vi "intersect circle.vi"(1 "max dist":dbl=40.0, 2 "R":dbl[](array[numeric]), 3 "Look":dbl(slide) scale=3.2..-3.2, 4 "R pos":dbl[](array[numeric]), 5 "py":dbl[](array[numeric]), 6 "px":dbl[](array[numeric])) -> (0 "Dist":dbl)   [LabVIEW 2009]
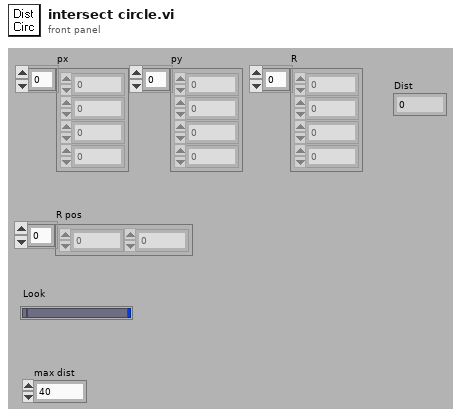
[diagram p1: front panel]
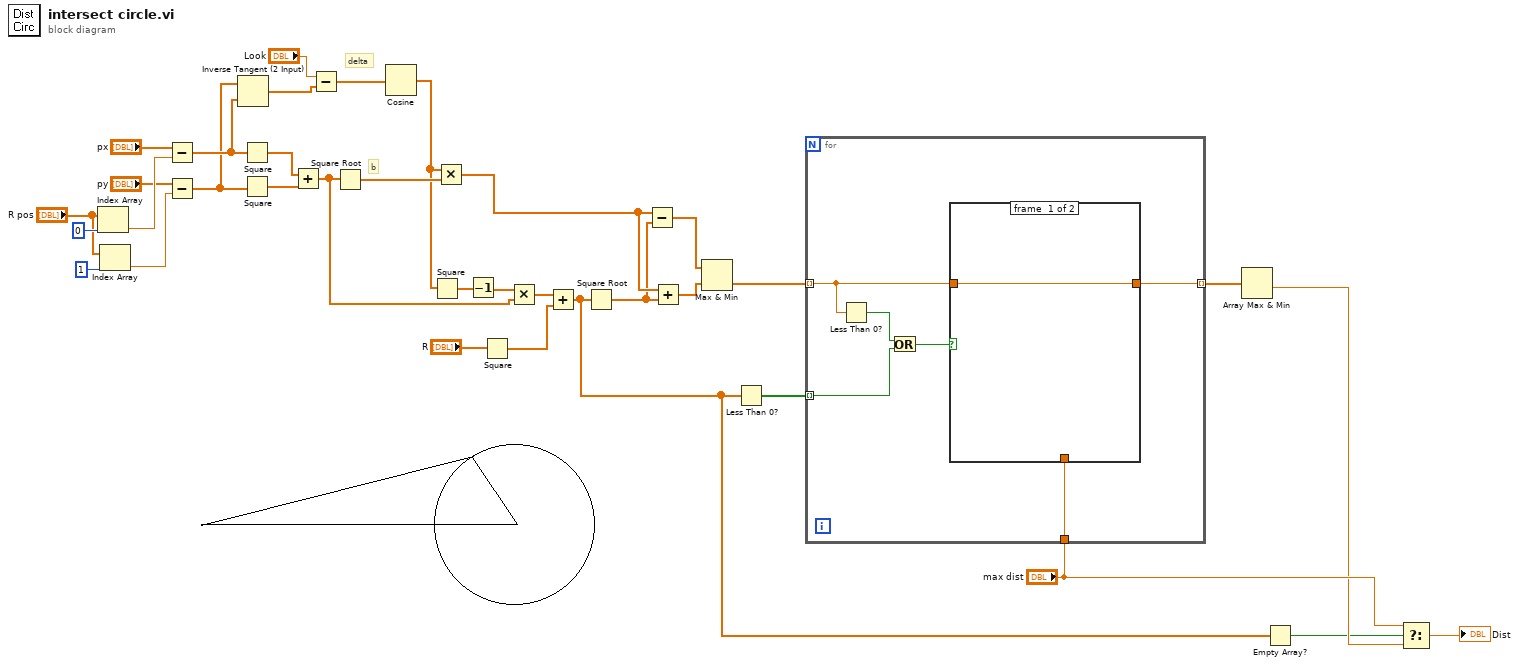
[diagram p0: block diagram]
diagram:
  # "b"
  # "delta"
  n1 = Index Array(array="R pos", index=0) -> (element=w31:dbl)
  n2 = Index Array(array="R pos", index=1) -> (element=w30:dbl)
  n3 = Subtract(x="px", y=w31) -> (x-y=w24:dbl[])
  n4 = Subtract(x="py", y=w30) -> (x-y=w23:dbl[])
  n5 = Inverse Tangent (2 Input)(1:w24, 2:w23) -> (0:w28:dbl[])
  n6 = Square(x=w24) -> (x^2=w21:dbl[])
  n7 = Square(x=w23) -> (x^2=w22:dbl[])
  n8 = Add(x=w21, y=w22) -> (x+y=w15:dbl[])
  n9 = Subtract(x="Look", y=w28) -> (x-y=w27:dbl[])
  n10 = Square Root(x=w15) -> (sqrt(x)=w19:dbl[])
  n11 = Cosine(x=w27) -> (cos(x)=w18:dbl[])
  n12 = Square(x=w18) -> (x^2=w17:dbl[])
  n13 = Multiply(x=w18, y=w19) -> (x*y=w12:dbl[])
  n14 = Decrement(x=w17) -> (x-1=w16:dbl[])
  n15 = Square(x="R") -> (x^2=w13:dbl[])
  n16 = Multiply(x=w16, y=w15) -> (x*y=w14:dbl[])
  n17 = Add(x=w14, y=w13) -> (x+y=w2:dbl[])
  n18 = Square Root(x=w2) -> (sqrt(x)=w11:dbl[])
  n19 = Subtract(x=w12, y=w11) -> (x-y=w10:dbl[])
  n20 = Add(x=w12, y=w11) -> (x+y=w9:dbl[])
  n21 = Max & Min(x=w10, y=w9) -> (min(x,y)=w7:dbl[])  [unwired: 1 out]
  n22 = Less Than 0?(x=w2) -> (x < 0?=w8:bool[])
  n23 = for {
    tunnel: w8 -> [w37] mode=indexing
    tunnel: w7 -> [w39] mode=indexing
    tunnel: [w40] -> w6 mode=indexing
    tunnel: "max dist" -> [w35]
    n24 = Less Than 0?(x=w39) -> (x < 0?=w38:bool)
    n25 = Or(x=w38, y=w37) -> (x .or. y?=w36:bool)
    n26 = case shown="True" w36 {
      tunnel: w39 -> [w41 _]
      tunnel: [w41 w42] -> w40
      tunnel: w35 -> [_ w42]
      frame #0 {
      }
      frame #1 {
      }
    }
  }
  n27 = Array Max & Min(array=w6) -> (min value=w4:dbl)  [unwired: 3 out]
  n28 = Empty Array?(array=w2) -> (empty?=w1:bool)
  n29 = Select(t="max dist", s=w1, f=w4) -> (s? t:f=→"Dist":dbl)
